vi "test Set ObjectType_2.vi"(11 "Test Entry":refnum<class "Test Object Entry.lvclass">) -> (0 "error out":errorcluster, 3 "Test Entry":refnum<class "Test Object Entry.lvclass">)   [LabVIEW 2020, in "Test Object Entry.lvclass"]
uses:
  Test Object Entry.lvclass
  Test Object Entry.lvclass/Test Object Entry.ctl
  source/Object Entry/Object Entry.lvclass
  source/Typedefs/Object Type.ctl
  source/CANopen.lvlib
  b059a695-546b-4a5a-ad62-058b8ba2a9b6.vi
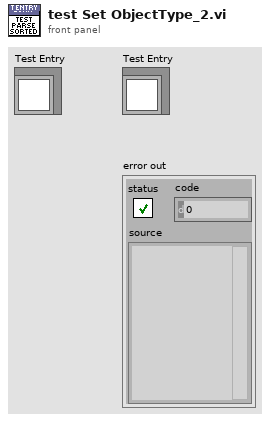
[diagram p1: front panel]
types:
  T1 = typedef "CANopen.lvlib/Object Type.ctl" = u8
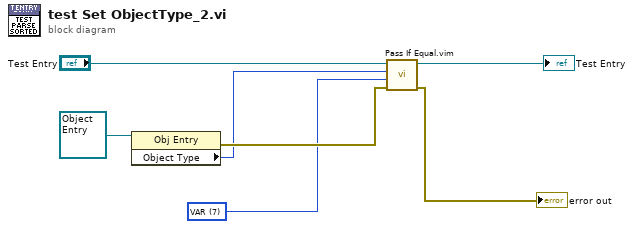
[diagram p0: block diagram]
diagram:
  w1 = T1 7 items=["NULL"=0, "DOMAIN"=2, "DEFTYPE"=5, "DEFSTRUCT"=6, "VAR"=7, "ARRAY"=8, "RECORD"=9] ("y")
  n1 = property class="Obj Entry"(reference=refnum<class "Object Entry.lvclass"> refnum ("EDS.lvlib:Object Type.lvclass")) -> (error out=w3:errorcluster, "Object Type"=w2:T1)  [unwired: 1 in, 1 out]
  n2 = call "Pass If Equal.vim"("error in (no error)"=w3, "Actual"=w1, "Expected"=w2, "LUnit Test Case In"="Test Entry") -> ("error out"=→"error out":errorcluster, "LUnit Test Case Out"=→"Test Entry":refnum<class "Test Object Entry.lvclass">)  [unwired: 6 in]
